vi "Destroy User Event - Stop.vi"(8 "error in (no error)":T1 caption="Fehler (Eingang, kein Fehler)", 11 "Benutzerereignis - Stopp":refnum<user-event>) -> (0 "error out":T1 caption="Fehler (Ausgang)")   [LabVIEW 2014, in "MyQH User Event - Stop.lvlib"]
doc: "Löscht das Benutzerereignis, auch wenn ein Fehler empfangen wird."
uses:
  MyQH User Event - Stop.lvlib
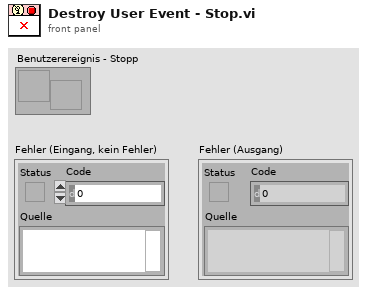
[diagram p1: front panel]
types:
  T1 = cluster{"Status":bool, "Code":i32, "Quelle":string}
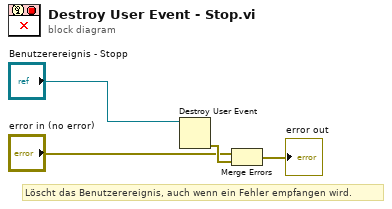
[diagram p0: block diagram]
diagram:
  # "Löscht das Benutzerereignis, auch wenn ein Fehler empfangen wird."
  n1 = Destroy User Event(user event="Benutzerereignis - Stopp") -> (error out=w3:errorcluster)  [unwired: 1 in]
  n2 = Merge Errors("error in (no error)", w3) -> (→"error out":errorcluster)
